vi "Close.vi"(8 "error in":errorcluster, 11 "Pressure Setpoint in":refnum<class "Pressure Setpoint.lvclass">) -> (0 "error out":errorcluster, 3 "Pressure Setpoint out":refnum<class "Pressure Setpoint.lvclass">)   [LabVIEW 2023, in "Pressure Setpoint.lvclass"]
uses:
  Pressure Setpoint.lvclass
  Parents/Setpoint/Setpoint.lvclass
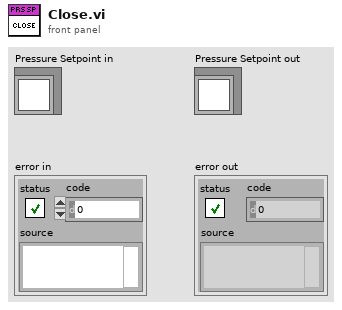
[diagram p1: front panel]
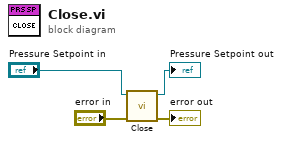
[diagram p0: block diagram]
diagram:
  n1 = call-parent "Close.vi"("error in"="error in", "Setpoint in"="Pressure Setpoint in") -> ("error out"=→"error out":errorcluster, "Setpoint out"=→"Pressure Setpoint out":refnum<class "Pressure Setpoint.lvclass">)  [unwired: 8 in]
